vi "Rawdata_Embdata_Analyer.vi"() -> ()   [LabVIEW 2020]
panel:
  out "Waveform Graph":u8[][](graph)
  out "Pre-Emb":u8[][](array[numeric]) format="%x"
  in  "stop":bool
  out "Progress":dbl(slide) scale=0.0..100.0
  out "error out":errorcluster
  out "Bytes per Frame":u32
  out "Total Frame Num":i64
  in  "RAWdata File Path":path
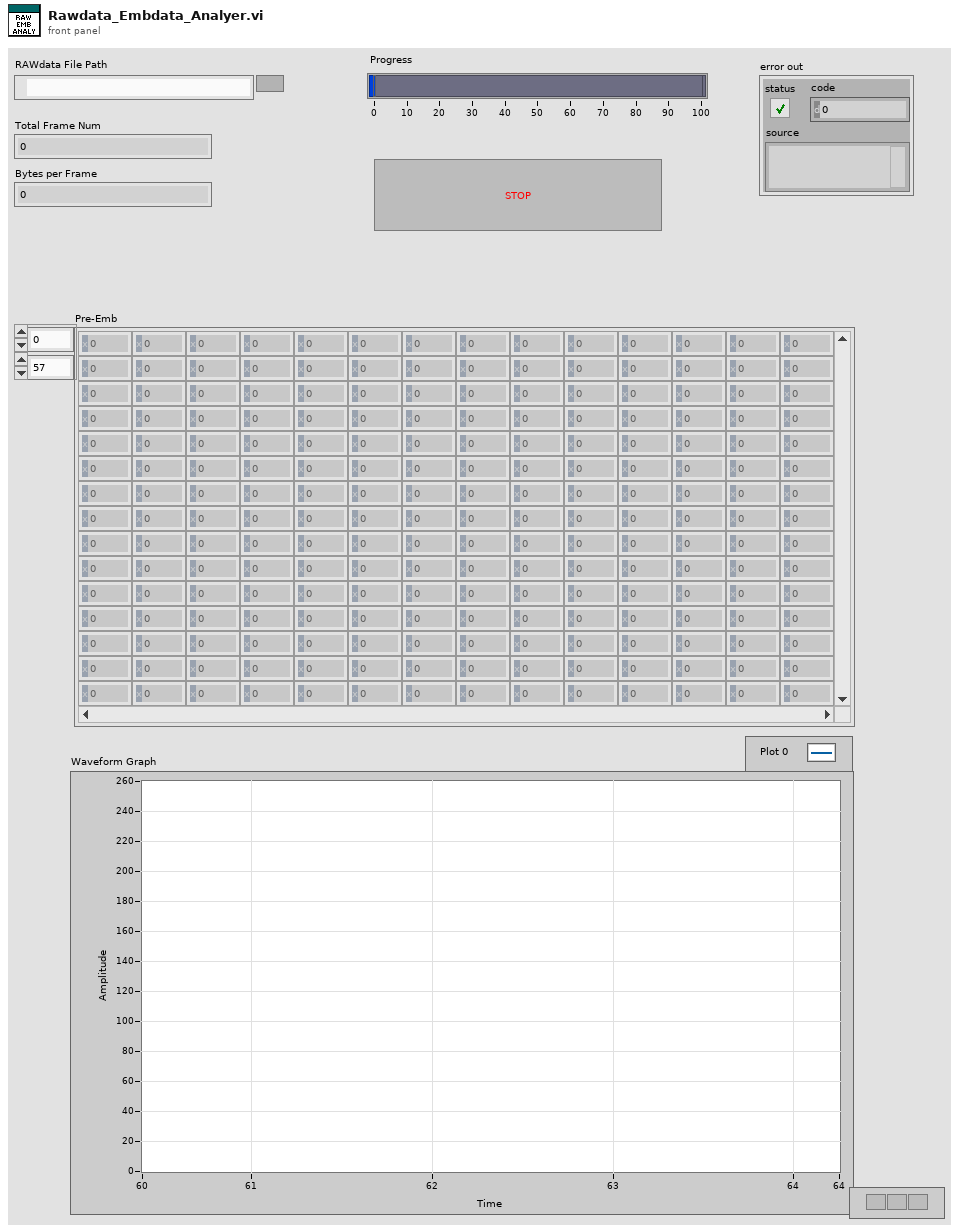
[diagram p1: front panel]
types:
  T1 = typedef "Image_Data_Config.ctl" = cluster{"Lines of Image Data":u16, "Bytes per Even Line":u16, "Bytes per Odd Line":u16, "Image Data Type":u8, "Total Image Data Block Size":u32, "Image Data Block Offset":u32}
  T2 = typedef "Image_EBD_Config.ctl" = cluster{"Lines of Pre-EBD Data":u16, "Lines of Post-EBD Data":u16, "Total EBD Block Size":u32, "Pre-EBD Block Offset ":u32, "Post-EBD Block Offset ":u32}
  T3 = enum16{"big-endian, network order", "native, host order", "little-endian"}
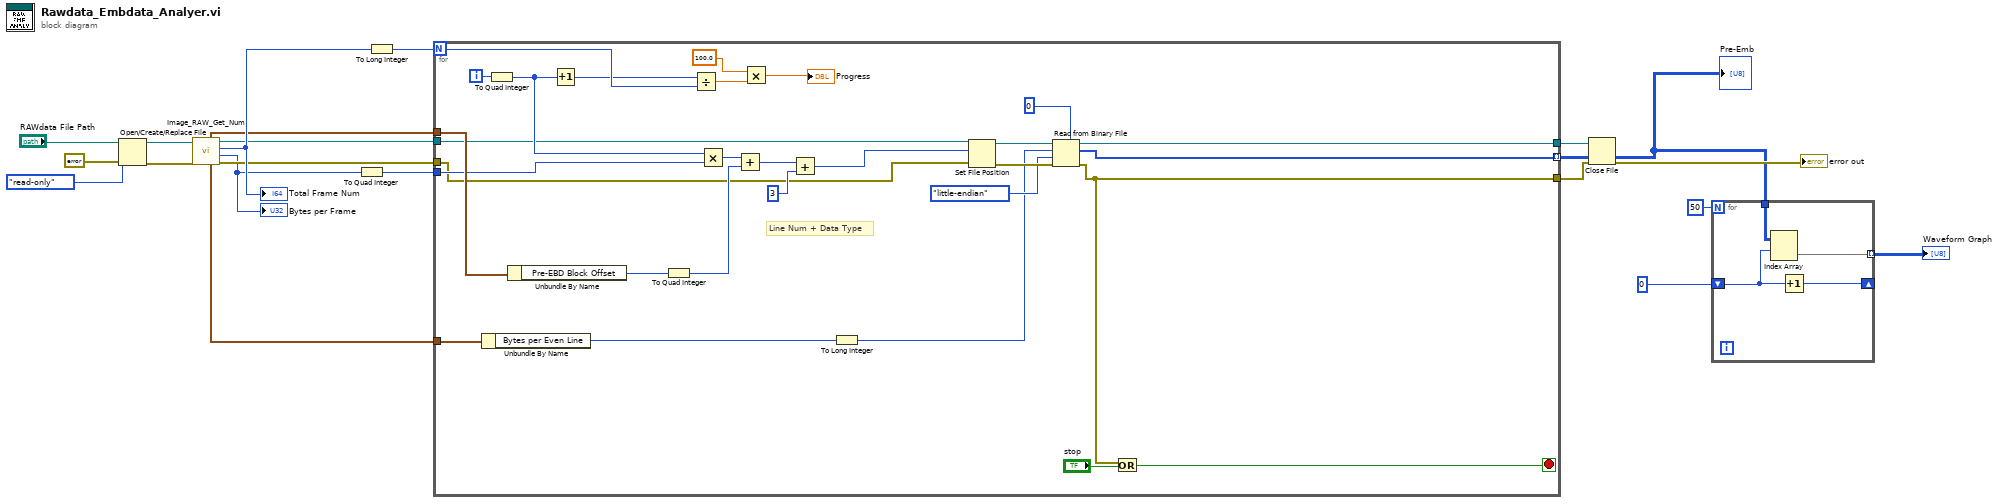
[diagram p0: block diagram]
diagram:
  n1 = Open/Create/Replace File(file path (use dialog)="RAWdata File Path", error in=errorcluster {"status"=FALSE, "code"=0, "source"=""}, access (0:read/write)=enum16{"read/write", "read-only", "write-only"}."read-only") -> (refnum out=w19:refnum<file>, error out=w18:errorcluster)  [unwired: 3 in, 1 out]
  n2 = call "Image_RAW_Get_Num.vi"("error in (no error)"=w18, "RAW refnum In"=w19) -> ("error out"=w14:errorcluster, "Bytes per Frame"=w10:u32, "Total Frame Num"=w16:i64, "RAW refnum Out"=w12:refnum<file>, "Image Data Config"=w8:T1, "EBD Config"=w11:T2)  [unwired: 4 in]
  "Total Frame Num" <- w16
  "Bytes per Frame" <- w10
  n3 = To Quad Integer(1:w10) -> (0:w9:i64)
  n4 = To Long Integer(number=w16) -> (32bit integer=w15:i32)
  n5 = for {
    N: w15 -> [w45]
    tunnel: w14 -> [w31]
    tunnel: w12 -> [w32]
    tunnel: w11 -> [w41]
    tunnel: w9 -> [w39]
    tunnel: w8 -> [w35]
    tunnel: [w21] -> w6
    tunnel: [w23] -> w2 mode=indexing
    tunnel: [w22] -> w7
    i -> [w49]
    stop <- w43 stop-if-true
    # "Line Num + Data Type"
    n6 = Unbundle By Name(w35) -> ("Bytes per Even Line"=w26:u16)
    n7 = To Quad Integer(1:w49) -> (0:w40:i64)
    n8 = Unbundle By Name(w41) -> ("Pre-EBD Block Offset"=w37:u32)
    n9 = Increment(x=w40) -> (x+1=w42:i64)
    n10 = To Quad Integer(1:w37) -> (0:w36:i64)
    n11 = Divide(x=w42, y=w45) -> (x/y=w47:dbl)
    n12 = Multiply(x=w40, y=w39) -> (x*y=w38:i64)
    n13 = Add(x=w38, y=w36) -> (x+y=w34:i64)
    n14 = Multiply(x=100.0, y=w47) -> (x*y=→"Progress":dbl)
    n15 = Add(x=w34, y=i64 3) -> (x+y=w30:i64)
    n16 = To Long Integer(number=w26) -> (32bit integer=w24:i32)
    n17 = Set File Position(offset (in bytes) (0)=w30, refnum=w32, error in=w31) -> (refnum out=w29:refnum<file>, error out=w28:errorcluster)  [unwired: 1 in]
    n18 = Read from Binary File(5:u8 0, 8:w28, 9:T3."little-endian" ("byte order (0:big-endian, network order)"), 10:w24, 11:w29) -> (0:w21:errorcluster, 2:w23:u8[], 3:w22:refnum<file>)  [unwired: 1 in, 1 out]
    n19 = Or(x=w21, y="stop") -> (x .or. y?=w43:bool)
  }
  "Pre-Emb" <- w2
  n20 = Close File(refnum=w7, error in=w6) -> (error out=→"error out":errorcluster)  [unwired: 1 out]
  n21 = for {
    N: 50 -> [_]
    shift-right: [w51] -> _
    shift-left: 0 -> [w52]
    tunnel: w2 -> [w53]
    tunnel: [w50] -> w1 mode=indexing
    n22 = Index Array(array=w53, index (row)=w52) -> (element=w50:u8[])  [unwired: 1 in]
    n23 = Increment(x=w52) -> (x+1=w51:i32)
  }
  "Waveform Graph" <- w1
